vi "001_Siemens S7 Series.vi"(11 "Queue Ref":T1={"UI"=refnum, "Message"=refnum, "Data"=refnum, "Caller"=refnum, "Name"="000 Common", "Data Path"=path "D:/NBT/01-Project/02-Processing/NBT-TestPlatform V2/NBT-TestPlatform V2.0.3/Config/NBT/NBT_V1.0.0/Project/0001_HZKD_ST01/00_DataSource/001_PLC/01_PLC", "Class Path"=path "", "SubPanel"=refnum, "Project Name"="", "MNT"="", "Title"="", "Data Source"=refnum, "Queue List"={}, "VI"=refnum, "UE"=refnum}) -> ()   [LabVIEW 2020]
doc: "S7"
uses:
  Alin/QMH/000 Module Data Type.ctl
  Alin/QMH/Queue Message.ctl
  9999 SubVI/Global/Data Global/SDQ Data Type.ctl
panel:
  out "Delay":u32 format="%.0f ms"
  out "QN":i32
  out "Data":string[][](table)
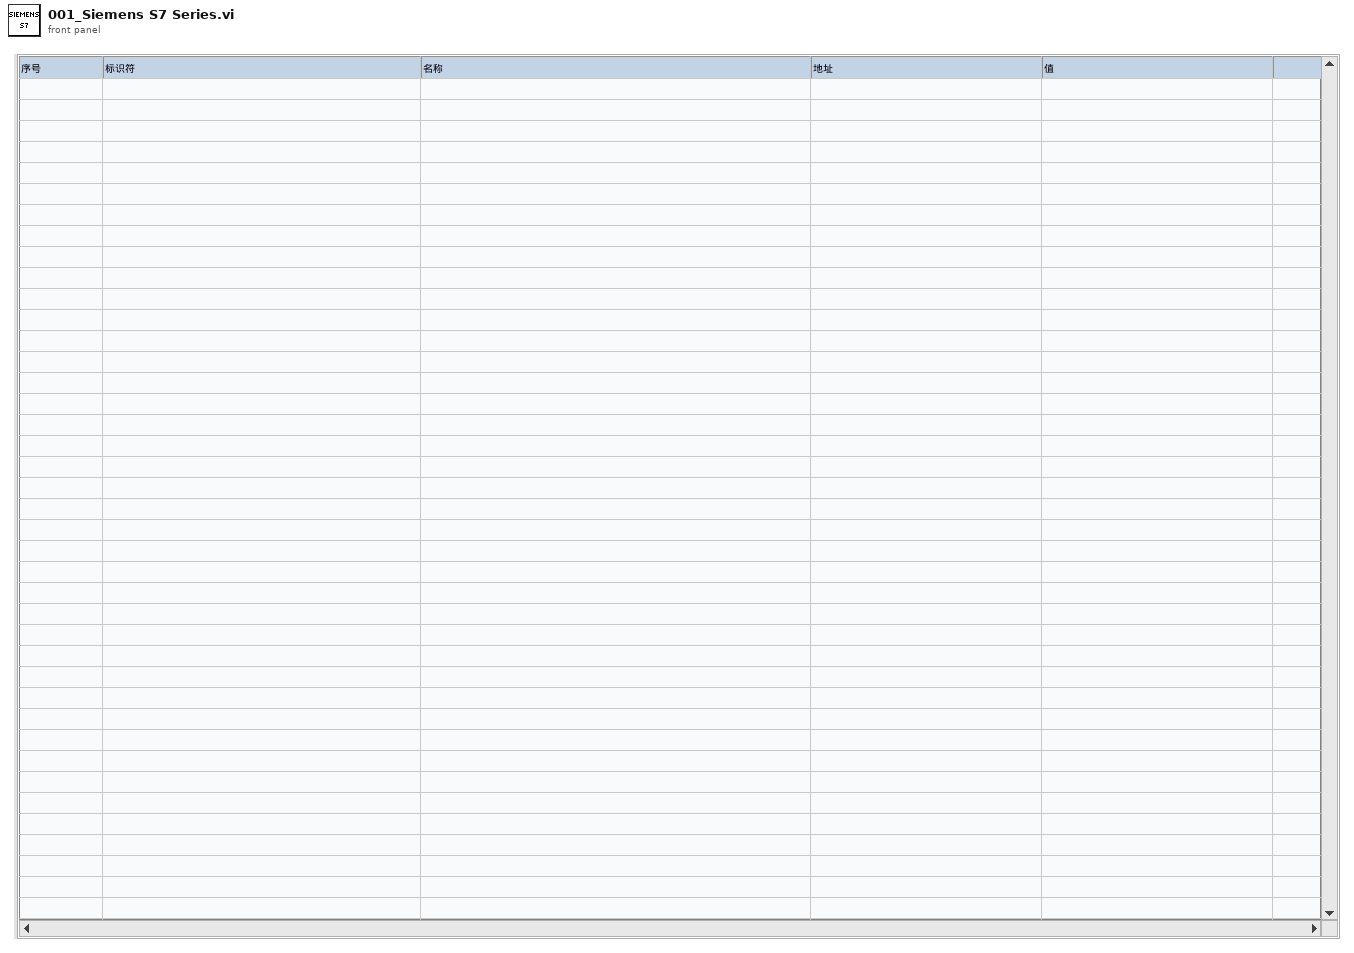
[diagram p1: front panel]
types:
  T1 = typedef "000 Module Data Type.ctl" = cluster{"UI":refnum<queue>, "Message":refnum<queue>, "Data":refnum<queue>, "Caller":refnum<queue>, "Name":string, "Data Path":path, "Class Path":path, "SubPanel":refnum<vi>, "Project Name":string, "MNT":string, "Title":string, "Data Source":refnum<queue>, "Queue List":map{string, refnum<queue>}, "VI":refnum<vi>, "UE":refnum<user-event>}
  T2 = typedef "SDQ Data Type.ctl" = cluster{"CAN Length":string, "CAN Name":string, "CAN ID":string, "CAN Type":string, "Test Item":string, "Byte Order":string, "Instruction":string, "Control Type":string, "Group":string, "Offset":dbl, "Coefficient":dbl, "Write Enable":bool, "Lable Type":string, "Key?":string, "Set Value":string, "Upper":dbl, "Lower":dbl, "Unit":string, "Formula":string, "Test Item Type":string, "Length":i32, "Address":string, "Name":string, "Identifier":string, "Data Type":string, "Enumerate?":string, "Enumerate List":string, "Data":string, "Source":string}
  T3 = cluster{"Read Data":map{string, string}, "Open?":bool, "Start?":bool, "Queue Ref":T1, "Data":map{string, T2}, "Data List":T2[], "PLC":cluster{"IP Address":string, "PLC":refnum<k5>, "Open?":bool, "Heart Beat":i32}, "Data1":map{string, cluster{"Data Type":enum16{"I", "Q", "M", "D", "Count", "Timer"}, u16, "Data":u8[], cluster{"Min":u16, u16}}}, "Source Data":string[][]}
  T4 = enum16{"S7-300/400/1200/1500", "S7-200", "S7-200Smart"}
  T5 = map{string, cluster{"Data Type":enum16{"I", "Q", "M", "D", "Count", "Timer"}, u16, "Data":u8[], cluster{"Min":u16, u16}}}
  T6 = cluster{"Data Type":enum16{"I", "Q", "M", "D", "Count", "Timer"}, u16, "Data":u8[], cluster{"Min":u16, u16}}
  T7 = cluster{"Name":string, "Read Data":map{string, string}}
  T8 = typedef "eventvkey.ctl" = enum16{"ASCII", "Enter", "Return", "Shift", "Ctrl", "Alt", "Cmd", "Opt", "Caps", "NumLock", "Clear", "Break", "Up", "Down", "Left", "Right", "Insert", "Delete", "Home", "End", "PageUp", "PageDown", "Escape", "Help", "Pause", "ScrollLock", "F1", "F2", "F3", "F4", "F5", "F6", "F7", "F8", "F9", "F10", "F11", "F12", "F13", "F14", "F15", "F16", "F17", "F18", "F19", "F20", "F21", "F22", "F23", "F24", "Play", "VolumeUp", "VolumeDown", "Mute", "Two Byte Char"}
  T9 = cluster{"Shift":bool, "Ctrl":bool, "Alt":bool, "Cmd":bool, "Opt":bool}
  T10 = cluster{"Queue List":map{string, refnum<queue>}, "Active Panel":string, "Queue Ref":T1}
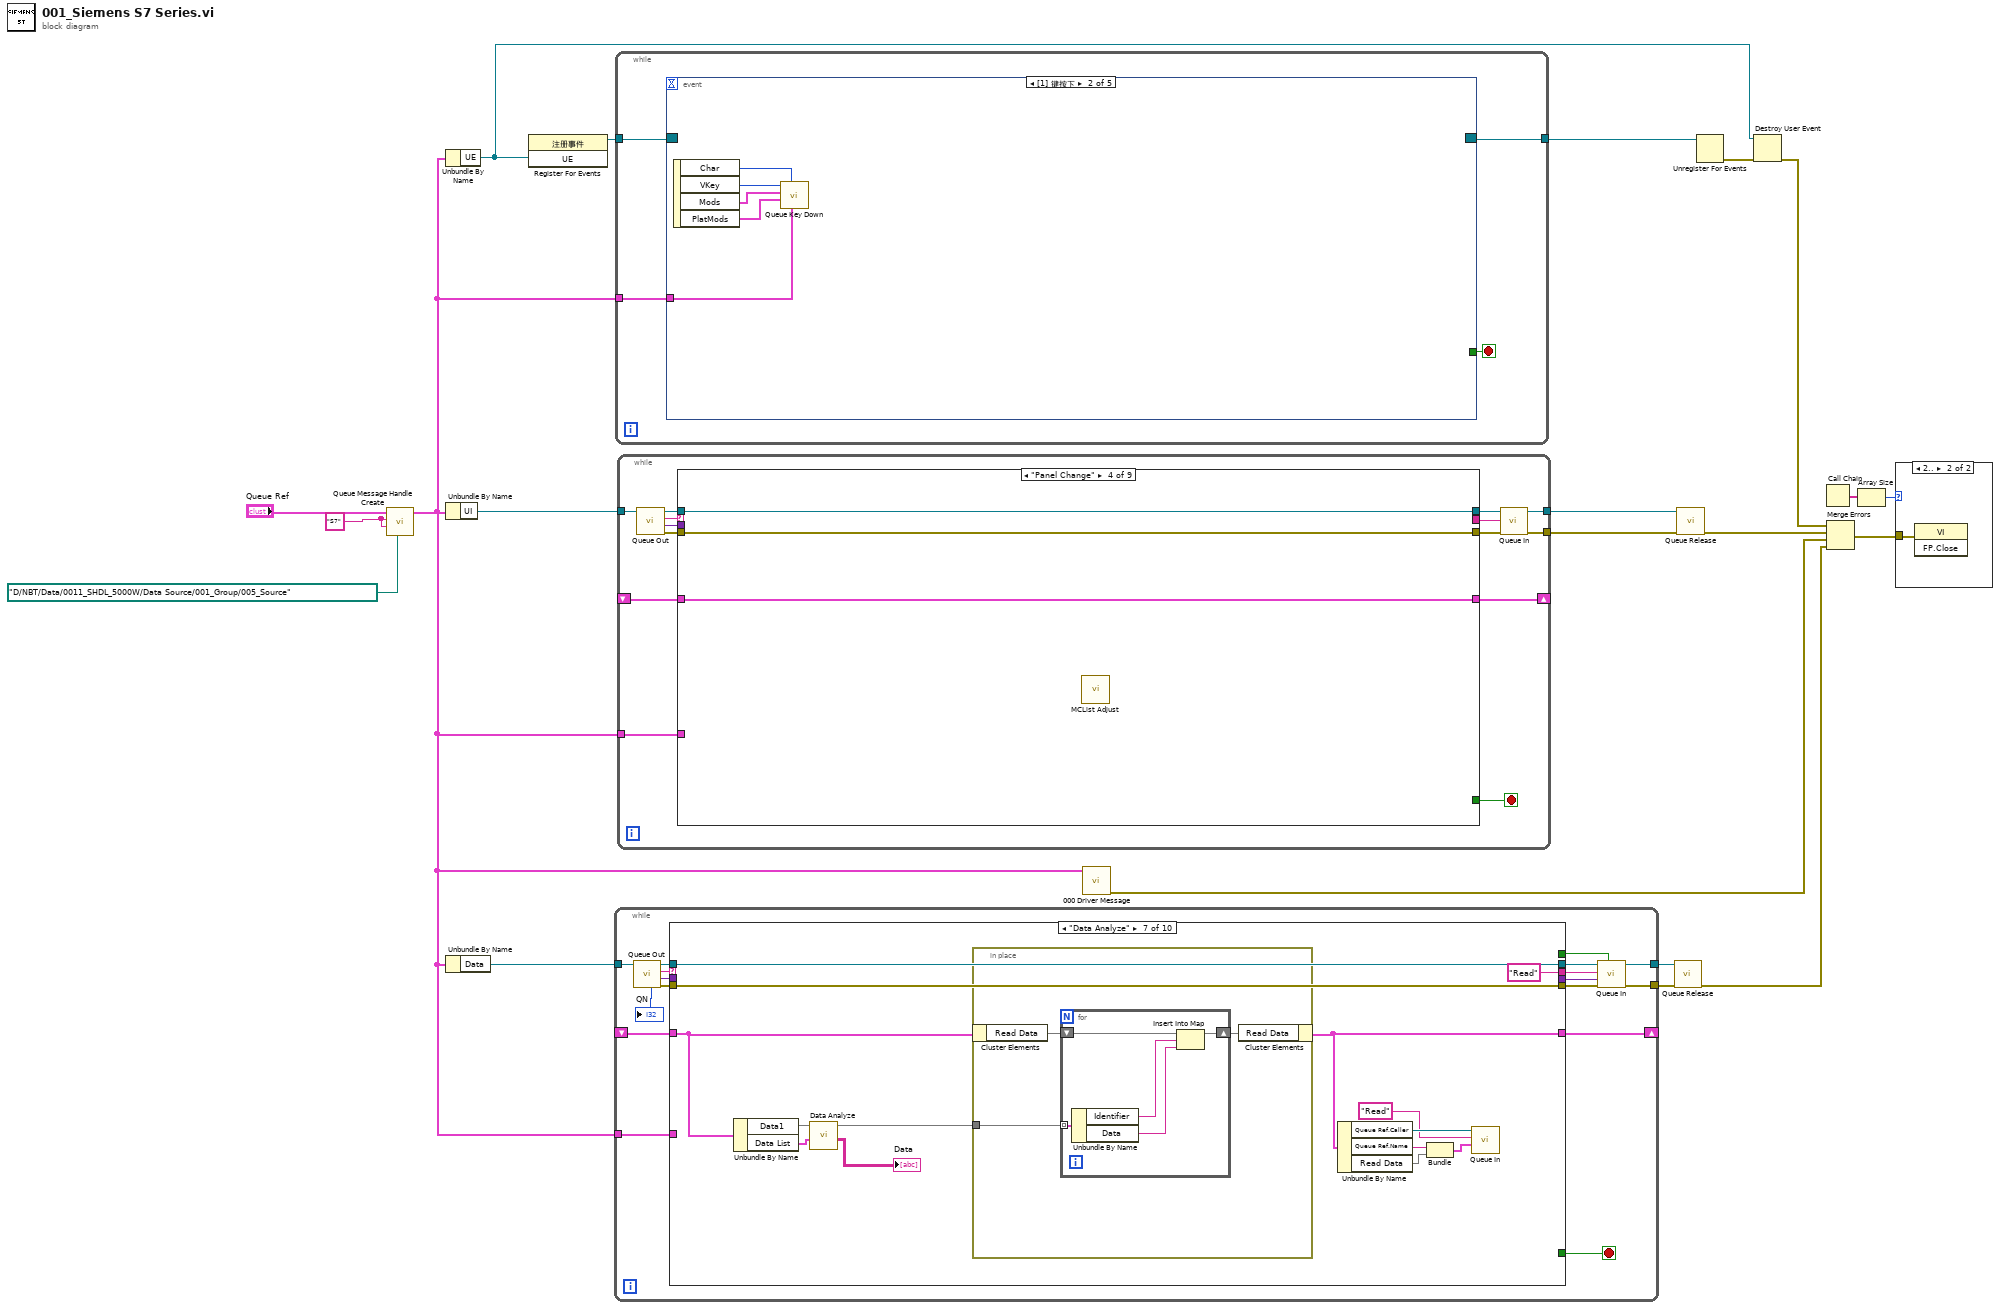
[diagram p0: block diagram]
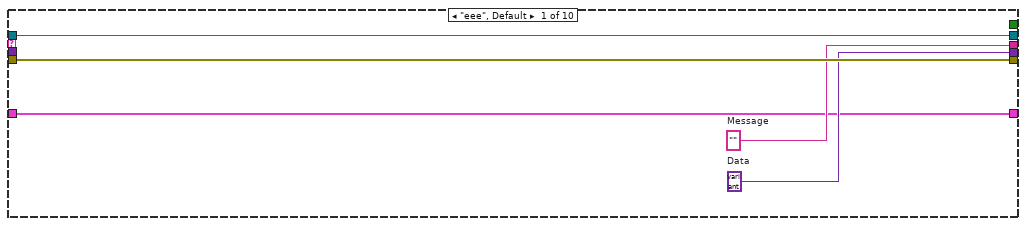
[diagram p2: hidden frame]
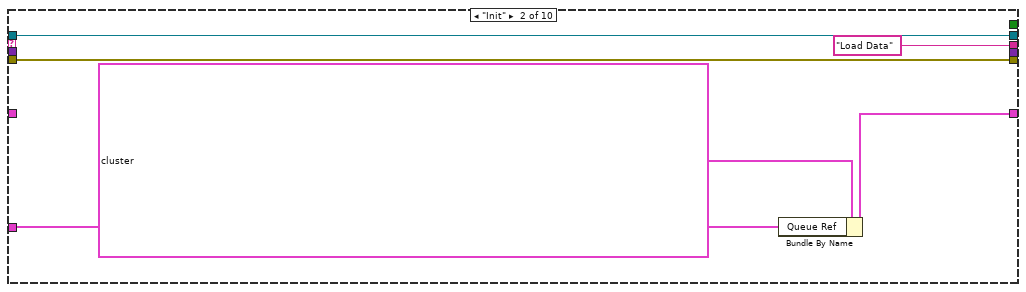
[diagram p3: hidden frame]
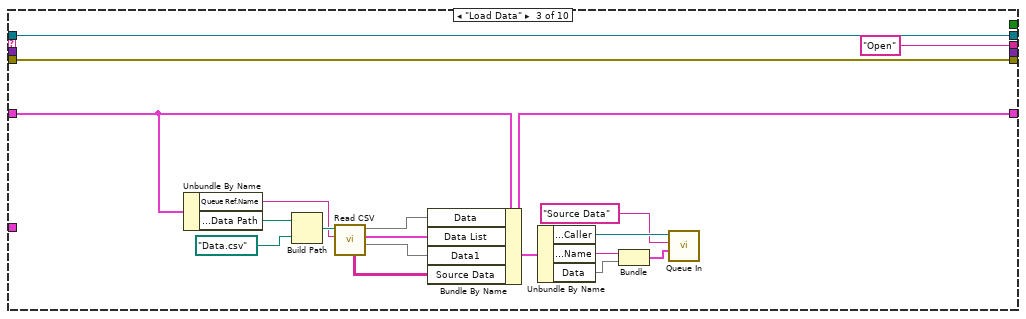
[diagram p4: hidden frame]
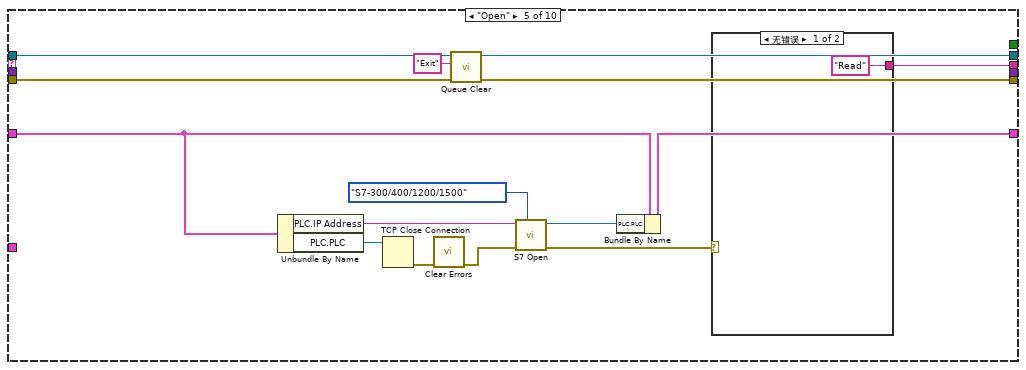
[diagram p6: hidden frame]
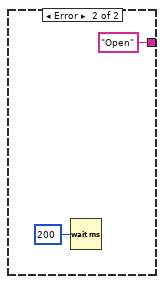
[diagram p7: hidden frame]
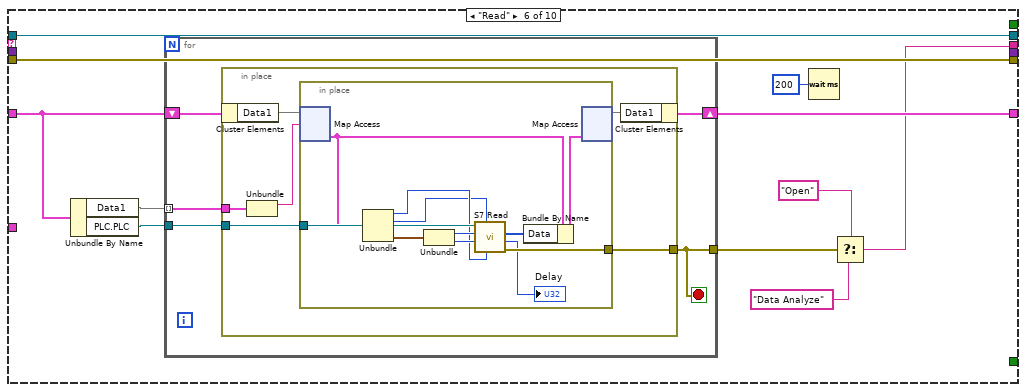
[diagram p8: hidden frame]
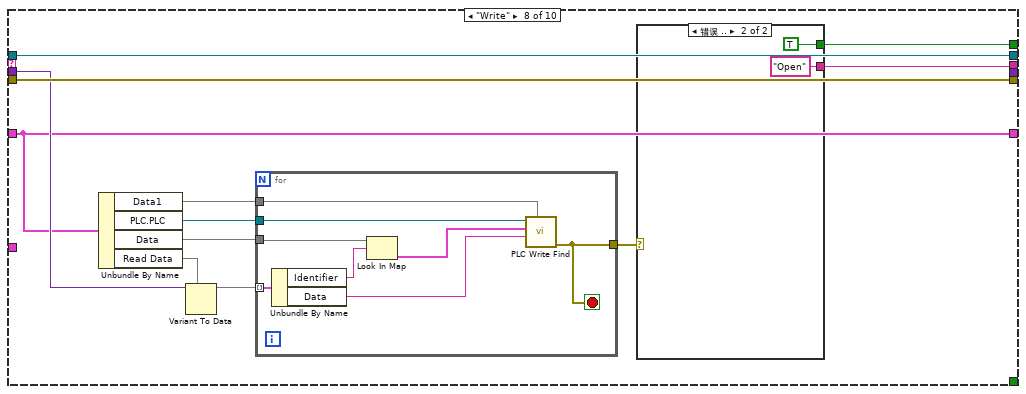
[diagram p9: hidden frame]
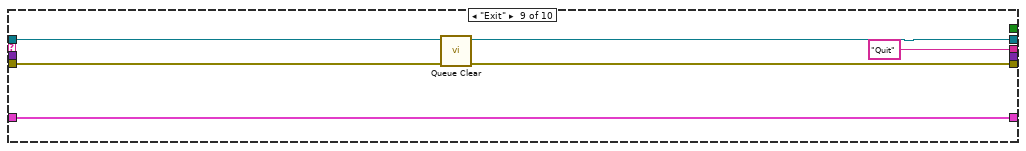
[diagram p11: hidden frame]
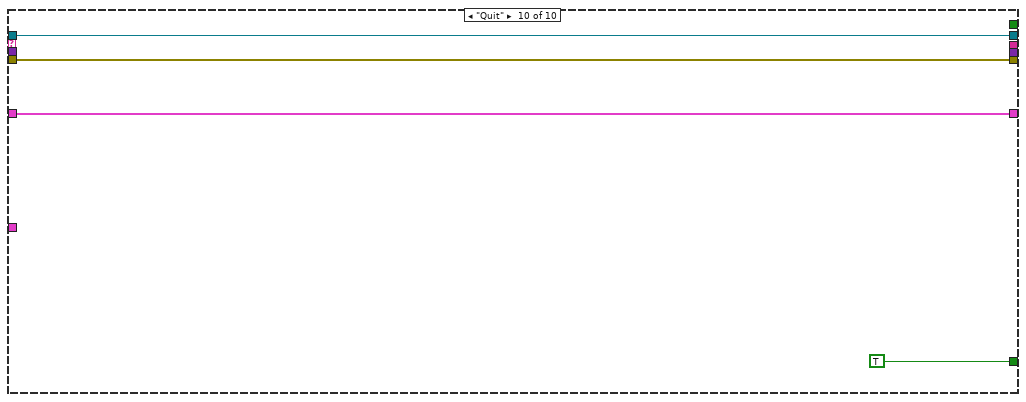
[diagram p12: hidden frame]
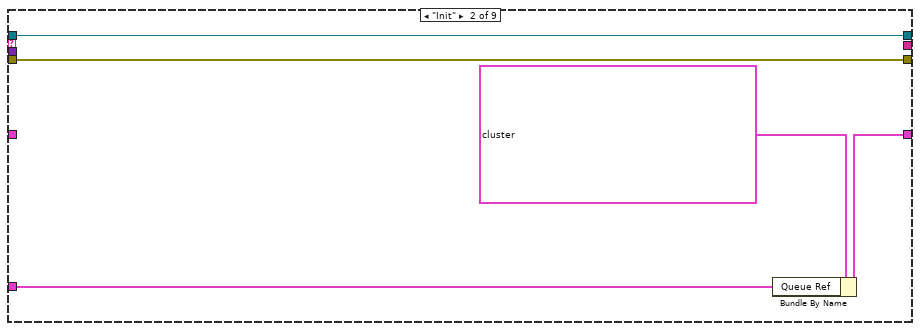
[diagram p15: hidden frame]
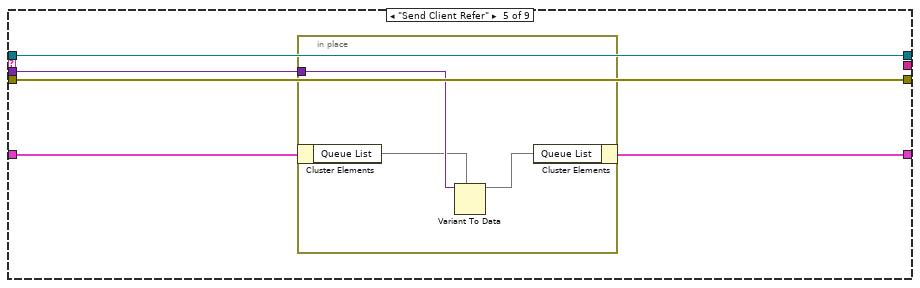
[diagram p17: hidden frame]
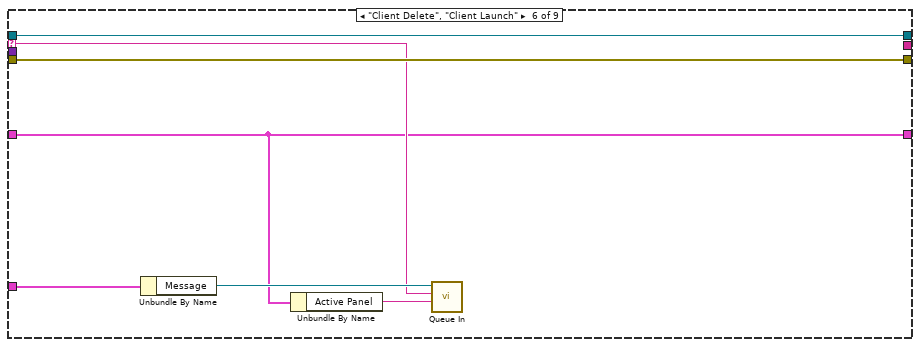
[diagram p18: hidden frame]
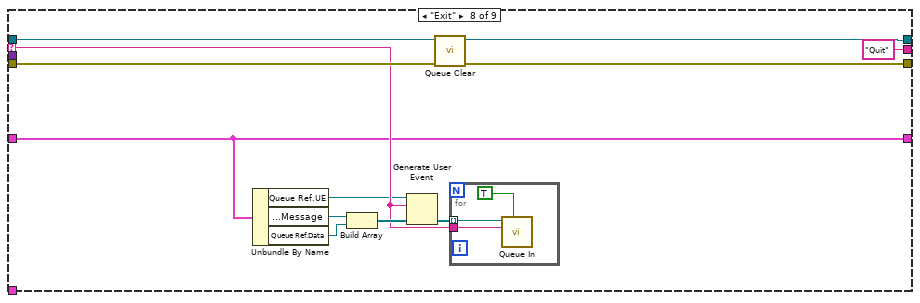
[diagram p20: hidden frame]
diagram:
  w1 = "S7" ("Title")
  n1 = call "Queue Message Handle Create.vi"("Data Path"=path "D:/NBT/Data/0011_SHDL_5000W/Data Source/001_Group/005_Source", "Name"=w1, "Title"=w1, "Queue Ref In"="Queue Ref") -> ("Queue Ref Out"=w4:T1)  [unwired: 6 in, 1 out]
  n2 = Unbundle By Name(w4) -> ("UE"=w3:refnum<user-event>)
  n3 = Unbundle By Name(w4) -> ("UI"=w11:refnum<queue>)
  n4 = Unbundle By Name(w4) -> ("Data"=w19:refnum<queue>)
  n5 = register-events(w3) -> (reference out=w6:refnum<event-registration>)  [unwired: 2 in, 1 out]
  n6 = while {
    tunnel: w19 -> [w34]
    tunnel: [w31] -> w17
    tunnel: [w30] -> w18
    shift-right: [w24] -> _
    shift-left: _ -> [w26]
    tunnel: w4 -> [w25]
    stop <- w38 stop-if-true
    n7 = call "Queue Out.vi"("Queue In"=w34) -> ("error out"=w37:errorcluster, "Data"=w35:variant, "Message"=w36:string, "Queue Out"=w33:refnum<queue>, "Queue NUmber"=→"QN":i32)  [unwired: 6 in]
    n8 = case shown="\"Data Analyze\"" w36 {
      tunnel: w33 -> [w43 w49 w67 w70 w75 w99 w135 w155 w170 w174]
      tunnel: w37 -> [w42 w48 w66 w69 w85 w98 w134 w154 w168 w175]
      tunnel: [w43 w49 w67 w70 w74 w99 w135 w155 w169 w174] -> w32
      tunnel: [w42 w48 w66 w69 w76 w98 w134 w154 w167 w175] -> w29
      tunnel: [w41 "Load Data" ("Message") "Open" ("Message") _ w71 w90 "Read" ("f") w145 "Quit" _] -> w28
      tunnel: [_ _ _ _ _ _ _ _ _ TRUE] -> w38
      tunnel: [w40 _ _ _ _ _ _ _ _ _] -> w27
      tunnel: w35 -> [_ _ _ _ _ _ _ w153 _ _]
      tunnel: [w39 w46 w54 w68 w78 w91 w127 w152 w166 w172] -> w24
      tunnel: w26 -> [w39 _ w65 w68 w79 w92 w130 w152 w166 w172]
      tunnel: w25 -> [_ w45 _ _ _ _ _ _ _ _]
      tunnel: [_ _ _ _ _ _ _ w144 _ _] -> w22
      frame "eee", Default {
        w40 = variant  # Data
        w41 = ""  # Message
      }
      frame "Init" {
        n9 = Bundle By Name(cluster=T3 {"Read Data"={}, "Open?"=FALSE, "Start?"=FALSE, "Queue Ref"={"UI"=refnum, "Message"=refnum, "Data"=refnum, "Caller"=refnum, "Name"="", "Data Path"=path "", "Class Path"=path "", "SubPanel"=refnum, "Project Name"="", "MNT"="", "Title"="", "Data Source"=refnum, "Queue List"={}, "VI"=refnum, "UE"=refnum}, "Data"={}, "Data List"=[], "PLC"={"IP Address"="192.168.0.3", "PLC"=refnum, "Open?"=FALSE, "Heart Beat"=0}, "Data1"={}, "Source Data"=[]}, "Queue Ref"=w45) -> (w46:T3)
      }
      frame "Load Data" {
        n10 = Unbundle By Name(w65) -> ("Queue Ref.Name"=w53:string, "Queue Ref.Data Path"=w64:path)
        n11 = Build Path(base path=w64, name or relative path=path "Data.csv" ("名称或相对路径")) -> (appended path=w62:path)
        n12 = call "Read CSV.vi"("Source"=w53, "Data Path"=w62) -> ("Data"=w58:T5, "Identifier List"=w60:T2[], "Identifiers Out"=w59:map{string, T2}, "Value Out"=w57:string[][])  [unwired: 2 in, 4 out]
        n13 = Bundle By Name(cluster=w65, "Data"=w59, "Data List"=w60, "Data1"=w58, "Source Data"=w57) -> (w54:T3)
        n14 = Unbundle By Name(w54) -> ("Queue Ref.Caller"=w56:refnum<queue>, "Queue Ref.Name"=w52:string, "Data"=w51:map{string, T2})
        n15 = Bundle("Name"=w52, "Data"=w51) -> (w50:cluster{"Name":string, "Data":map{string, T2}})  [unwired: 1 in]
        n16 = call "Queue In.vi"("Data"=w50, "Message"="Source Data", "Queue In"=w56) -> ()  [unwired: 7 in, 2 out]
      }
      frame "====Driver====" {
      }
      frame "Open" {
        n17 = Unbundle By Name(w79) -> ("PLC.IP Address"=w84:string, "PLC.PLC"=w82:refnum<k5>)
        n18 = TCP Close Connection(connection ID=w82) -> (error out=w81:errorcluster)  [unwired: 2 in, 1 out]
        n19 = call <vilib>:"Clear Errors.vi"("error in (no error)"=w81) -> ("error out"=w80:errorcluster)  [unwired: 5 in, 1 out]
        n20 = call "Queue Clear.vi"("error in (no error)"=w85, "Filter"="Exit", "Queue In"=w75) -> ("error out"=w76:errorcluster, "Queue Out"=w74:refnum<queue>)  [unwired: 7 in]
        n21 = call "S7 Open.vi"("PLC type"=T4."S7-300/400/1200/1500", "Error In"=w80, "remote address"=w84) -> ("error out"=w72:errorcluster, "TCP Out"=w77:refnum<k5>)  [unwired: 6 in, 1 out]
        n22 = Bundle By Name(cluster=w79, "PLC.PLC"=w77) -> (w78:T3)
        n23 = case shown="无错误" w72 {
          tunnel: ["Read" "Open"] -> w71
          frame No Error {
          }
          frame Error {
            n24 = Wait (ms)(milliseconds to wait=u32 200 ("等待时间（毫秒）")) -> ()  [unwired: 1 out]
          }
        }
      }
      frame "Read" {
        n25 = Unbundle By Name(w92) -> ("Data1"=w96:T5, "PLC.PLC"=w95:refnum<k5>)
        n26 = for {
          tunnel: w95 -> [w104]
          tunnel: w96 -> [w100] mode=indexing
          shift-right: [w102] -> w91
          shift-left: w92 -> [w103]
          tunnel: [w101] -> w97
          stop <- w101 stop-if-true
          n27 = in-place {
            in-place-border: w104 -> [w110]
            in-place-border: [w109] -> w101
            in-place-border: w100 -> [w107]
            n28 = in-place-cluster #1(w103) -> ("Data1"=w108:T5)
            n29 = Unbundle(w107) -> ("Data Type"=w106:string)  [unwired: 1 out]
            n30 = in-place {
              in-place-border: w110 -> [w121]
              in-place-border: [w117] -> w109
              n31 = in-place-map #2(w108, w106) -> (w114:T6)  [unwired: 1 in, 1 out]
              n32 = Unbundle(w114) -> ("Data Type"=w112:enum16{"I", "Q", "M", "D", "Count", "Timer"}, w111:u16, w113:cluster{"Min":u16, u16})  [unwired: 1 out]
              n33 = Unbundle(w113) -> ("Min"=w119:u16, w118:u16)
              n34 = call "S7 Read.vi"("Data Type"=w112, "DB.NO."=w111, "count"=w118, "StartByteAddr"=w119, "TCP In"=w121) -> ("error out"=w117:errorcluster, "Delay"=→"Delay":u32, "Read Data"=w120:u8[])  [unwired: 3 in, 1 out]
              n35 = Bundle By Name(cluster=w114, "Data"=w120) -> (w116:T6)
              n36 = in-place-map #2(w116) -> (w105:T5)  [unwired: 1 in, 2 out]
            }
            n37 = in-place-cluster #1("Data1"=w105) -> (w102:T3)
          }
        }
        n38 = Wait (ms)(milliseconds to wait=u32 200 ("等待时间（毫秒）")) -> ()  [unwired: 1 out]
        n39 = Select(t="Open", s=w97, f="Data Analyze") -> (s? t:f=w90:string)
      }
      frame "Data Analyze" {
        n40 = Unbundle By Name(w130) -> ("Data1"=w132:T5, "Data List"=w133:T2[])
        n41 = call "Data Analyze.vi"("Identifier List"=w133, "Data"=w132) -> ("Data Out"=→"Data":string[][], "Send Data"=w131:map{string, string})  [unwired: 6 in, 2 out]
        n42 = in-place {
          in-place-border: w131 -> [w136]
          n43 = in-place-cluster #3(w130) -> ("Read Data"=w138:map{string, string})
          n44 = for {
            tunnel: w136 -> [w143] mode=indexing
            shift-right: [w139] -> w137
            shift-left: w138 -> [w142]
            n45 = Unbundle By Name(w143) -> ("Identifier"=w141:string, "Data"=w140:string)
            n46 = Insert Into Map(map in=w142, key=w141, value=w140) -> (map out=w139:map{string, string})  [unwired: 2 out]
          }
          n47 = in-place-cluster #3("Read Data"=w137) -> (w127:T3)
        }
        n48 = Unbundle By Name(w127) -> ("Queue Ref.Caller"=w129:refnum<queue>, "Queue Ref.Name"=w125:string, "Read Data"=w123:map{string, string})
        n49 = Bundle("Name"=w125, "Read Data"=w123) -> (w124:T7)  [unwired: 1 in]
        n50 = call "Queue In.vi"("Data"=w124, "Message"="Read", "Queue In"=w129) -> ()  [unwired: 7 in, 2 out]
      }
      frame "Write" {
        n51 = Unbundle By Name(w152) -> ("Data1"=w147:T5, "PLC.PLC"=w148:refnum<k5>, "Data"=w150:map{string, T2}, "Read Data"=w151:map{string, string})
        n52 = Variant To Data(type=w151, Variant=w153) -> (data=w149:map{string, string})  [unwired: 1 in, 1 out]
        n53 = for {
          tunnel: w149 -> [w164] mode=indexing
          tunnel: w150 -> [w165]
          tunnel: w148 -> [w162]
          tunnel: w147 -> [w159]
          tunnel: [w158] -> w146
          stop <- w158 stop-if-true
          n54 = Unbundle By Name(w164) -> ("Identifier"=w163:string, "Data"=w160:string)
          n55 = Look In Map(map=w165, key=w163) -> (value=w161:T2)  [unwired: 1 in, 1 out]
          n56 = call "PLC Write Find.vi"("Data1 In"=w159, "Data In"=w160, "Data"=w161, "PLC.PLC"=w162) -> ("error out"=w158:errorcluster)  [unwired: 7 in]
        }
        n57 = case shown="错误 .." w146 {
          tunnel: [_ "Open"] -> w145
          tunnel: [_ TRUE] -> w144
          frame No Error {
          }
          frame Error {
          }
        }
      }
      frame "Exit" {
        n58 = call "Queue Clear.vi"("error in (no error)"=w168, "Queue In"=w170) -> ("error out"=w167:errorcluster, "Queue Out"=w169:refnum<queue>)  [unwired: 8 in]
      }
      frame "Quit" {
      }
    }
    n59 = call "Queue In.vi"("First"=w22, "error in (no error)"=w29, "Data"=w27, "Message"=w28, "Queue In"=w32) -> ("error out"=w30:errorcluster, "Queue Out"=w31:refnum<queue>)  [unwired: 5 in]
  }
  n60 = while {
    tunnel: w6 -> [w179]
    tunnel: [w177] -> w7
    tunnel: w4 -> [w176]
    stop <- w178 stop-if-true
    n61 = event shown="[1] 键按下" {
      selector: w179 -> [_ _ _ _ _]
      dyn-events: [_ _ _ _ _] -> w177
      timeout: _ -> [_ _ _ _ _]
      tunnel: [_ _ _ w188 _] -> w178
      tunnel: w176 -> [_ w182 w187 _ w192]
      event Timeout {
        n62 = event-data() -> ()  [unwired: 1 in, 1 out]
      }
      event Key Down {
        n63 = event-data() -> ("Char"=w184:i16, "VKey"=w183:T8, "Mods"=w181:cluster{"Num Pad":bool, "Menu Key":bool}, "PlatMods"=w180:T9)  [unwired: 1 in]
        n64 = call "Queue Key Down.vi"("Queue Ref Out"=w182, "C"=w184, "Platform Key"=w180, "Group Key"=w181, "V Key"=w183) -> ()  [unwired: 6 in, 1 out]
      }
      event Panel Resize {
        n65 = event-data() -> ()  [unwired: 1 in, 1 out]
        n66 = Unbundle By Name(w187) -> ("Message"=w186:refnum<queue>)
        n67 = call "Queue In.vi"("Message"="Panel Change", "Queue In"=w186) -> ()  [unwired: 8 in, 2 out]
      }
      event User Event {
        n68 = event-data() -> ("Message"=w190:string)  [unwired: 1 in]
        n69 = Equal?(x=w190, y="Exit") -> (x = y?=w188:bool)
      }
      event Panel Close? {
        n70 = event-data() -> ()  [unwired: 1 in, 1 out]
        n71 = Unbundle By Name(w192) -> ("Message"=w191:refnum<queue>)
        n72 = Call Chain() -> (call chain=w195:string[])
        n73 = Array Size(array=w195) -> (size(s)=w194:i32)
        n74 = case shown="0, 默认" w194 {
          tunnel: ["Exit Prepare" ("Message") "Panel Hidden" ("Message")] -> w193
          frame 0, Default {
          }
          frame 2.. {
          }
        }
        n75 = call "Queue In.vi"("Message"=w193, "Queue In"=w191) -> ()  [unwired: 8 in, 2 out]
        n76 = event-data("Discard?"=TRUE ("放弃？")) -> ()  [unwired: 1 in, 1 out]
      }
    }
  }
  n77 = while {
    tunnel: w11 -> [w208]
    tunnel: [w205] -> w9
    tunnel: [w204] -> w10
    tunnel: w4 -> [w201]
    shift-right: [w200] -> _
    shift-left: _ -> [w199]
    stop <- w212 stop-if-true
    n78 = call "Queue Out.vi"("Queue In"=w208) -> ("error out"=w211:errorcluster, "Data"=w209:variant, "Message"=w210:string, "Queue Out"=w207:refnum<queue>)  [unwired: 6 in, 1 out]
    n79 = case shown="\"Panel Change\"" w210 {
      selector: w210 -> [_ _ _ _ _ w237 _ w249 _]
      tunnel: w207 -> [w215 w220 w223 w226 w231 w241 w244 w254 w261]
      tunnel: w211 -> [w214 w219 w222 w225 w230 w240 w243 w252 w262]
      tunnel: [w215 w220 w223 w226 w231 w241 w244 w253 w261] -> w206
      tunnel: [w214 w219 w222 w225 w230 w240 w243 w251 w262] -> w203
      tunnel: [_ _ _ _ _ _ _ "Quit" _] -> w202
      tunnel: [_ _ _ _ _ _ _ _ TRUE] -> w212
      tunnel: w209 -> [_ _ _ _ w227 _ _ _ _]
      tunnel: w201 -> [_ w216 _ _ _ w239 _ _ _]
      tunnel: [w213 w217 w221 w224 w228 w236 w242 w248 w259] -> w200
      tunnel: w199 -> [w213 _ w221 w224 w229 w236 w242 w248 w259]
      frame "eee", Default {
      }
      frame "Init" {
        n80 = Bundle By Name(cluster=T10 {"Queue List"={}, "Active Panel"="", "Queue Ref"={"UI"=refnum, "Message"=refnum, "Data"=refnum, "Caller"=refnum, "Name"="", "Data Path"=path "", "Class Path"=path "", "SubPanel"=refnum, "Project Name"="", "MNT"="", "Title"="", "Data Source"=refnum, "Queue List"={}, "VI"=refnum, "UE"=refnum}}, "Queue Ref"=w216) -> (w217:T10)
      }
      frame "====System====" {
      }
      frame "Panel Change" {
        n81 = call "MCList Adjust.vi"() -> ()  [unwired: 11 in, 1 out]
      }
      frame "Send Client Refer" {
        n82 = in-place {
          in-place-border: w227 -> [w233]
          n83 = in-place-cluster #4(w229) -> ("Queue List"=w232:map{string, refnum<queue>})
          n84 = Variant To Data(type=w232, Variant=w233) -> (data=w234:map{string, refnum<queue>})  [unwired: 1 in, 1 out]
          n85 = in-place-cluster #4("Queue List"=w234) -> (w228:T10)
        }
      }
      frame "Client Delete", "Client Launch" {
        n86 = Unbundle By Name(w239) -> ("Message"=w238:refnum<queue>)
        n87 = Unbundle By Name(w236) -> ("Active Panel"=w235:string)
        n88 = call "Queue In.vi"("Data"=w235, "Message"=w237, "Queue In"=w238) -> ()  [unwired: 7 in, 2 out]
      }
      frame "====User====" {
      }
      frame "Exit" {
        n89 = Unbundle By Name(w248) -> ("Queue Ref.UE"=w245:refnum<user-event>, "Queue Ref.Message"=w247:refnum<queue>, "Queue Ref.Data"=w246:refnum<queue>)
        n90 = Build Array(w247, w246) -> (w250:refnum<queue>[])
        n91 = Generate User Event(user event=w245, event data cluster=w249) -> ()  [unwired: 2 in, 2 out]
        n92 = call "Queue Clear.vi"("error in (no error)"=w252, "Queue In"=w254) -> ("error out"=w251:errorcluster, "Queue Out"=w253:refnum<queue>)  [unwired: 8 in]
        n93 = for {
          tunnel: w250 -> [w258] mode=indexing
          tunnel: w249 -> [w257]
          n94 = call "Queue In.vi"("First"=TRUE, "Message"=w257, "Queue In"=w258) -> ()  [unwired: 7 in, 2 out]
        }
      }
      frame "Quit" {
      }
    }
    n95 = call "Queue In.vi"("error in (no error)"=w203, "Message"=w202, "Queue In"=w206) -> ("error out"=w204:errorcluster, "Queue Out"=w205:refnum<queue>)  [unwired: 7 in]
  }
  n96 = call "000 Driver Message.vi"("Queue In"=w4) -> ("error out"=w20:errorcluster)  [unwired: 8 in, 2 out]
  n97 = call "Queue Release.vi"("error in (no error)"=w18, "Queue In"=w17) -> ("error out"=w21:errorcluster)  [unwired: 9 in]
  n98 = call "Queue Release.vi"("error in (no error)"=w10, "Queue In"=w9) -> ("error out"=w13:errorcluster)  [unwired: 9 in]
  n99 = Unregister For Events(event registration refnum=w7) -> (error out=w8:errorcluster)  [unwired: 1 in]
  n100 = Destroy User Event(user event=w3, error in=w8) -> (error out=w12:errorcluster)
  n101 = Call Chain() -> (call chain=w15:string[])
  n102 = Merge Errors(w12, w13, w20, w21) -> (w14:errorcluster)
  n103 = Array Size(array=w15) -> (size(s)=w16:i32)
  n104 = case shown="2.." w16 {
    tunnel: w14 -> [_ w263]
    frame 0, Default {
    }
    frame 2.. {
      n105 = invoke class="VI" method="FP.Close"(error in=w263) -> ()  [unwired: 2 in, 3 out]
    }
  }
